vi "CastByteArrayAndDispatchMsg.vi"(8 "error in (no error)":errorcluster, 10 "Raw Data":i8[](array[numeric]), 11 "DIMDemoClient in":refnum<class "DIMDemoClient.lvclass">) -> (0 "error out":errorcluster, 3 "DIMDemoClient out":refnum<class "DIMDemoClient.lvclass">)   [LabVIEW 2012, in "DimActorDemo.lvlib" / "DIMDemoClient.lvclass"]
doc: "Type cast byte array to G data with respect to type descriptor and dispatch message to self.\n\n<b>Needs to be overwitten by derived class.</b>"
uses:
  DIMDemoClient.lvclass
  <vilib>/ActorFramework/Actor/Actor.lvclass/Actor.ctl
  <vilib>/ActorFramework/Message Enqueuer/Message Enqueuer.lvclass/Message Enqueuer.ctl
  DIMDemoClient Messages/Update DemoService Msg/UpdateGUI DemoService Msg.lvclass/UpdateGUI DemoService Msg.ctl
  <vilib>/ActorFramework/Message Enqueuer/Init from Existing Queue.vi
  <vilib>/ActorFramework/Message Enqueuer/Enqueue.vi
  <vilib>/ActorFramework/Message Priority Queue/Priority Enqueue.vi
  <vilib>/ActorFramework/Message Enqueuer/Message Enqueuer.lvclass
  DIMDemoClient Messages/Update DemoService Msg/UpdateGUI DemoService Msg.lvclass
  <vilib>/ActorFramework/Actor/Actor.lvclass
  SVN/LV2009/GPL/lib.lib/DimLVEvent/LVDimInterface/LVDimInterface.lvlib
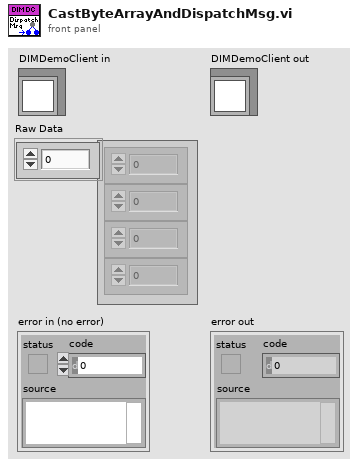
[diagram p1: front panel]
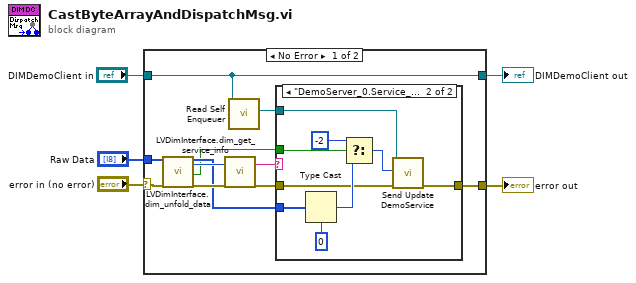
[diagram p0: block diagram]
diagram:
  n1 = case shown="No Error" "error in (no error)" {
    selector: "error in (no error)" -> [w7 w28]
    tunnel: "Raw Data" -> [w9 _]
    tunnel: [w8 w28] -> w4
    tunnel: "DIMDemoClient in" -> [w6 w27]
    tunnel: [w6 w27] -> w1
    frame No Error {
      n2 = call "LVDimInterface.dim_unfold_data.vi"("rawData"=w9, "error in (no error)"=w7) -> ("data"=w13:i8[], "callBackID"=w16:i32, "no link"=w10:bool, "error out"=w15:errorcluster)  [unwired: 14 in]
      n3 = call "LVDimInterface.dim_get_service_info.vi"("callBackID"=w16, "error in (no error)"=w15) -> ("serviceName"=w14:string, "error out"=w11:errorcluster)  [unwired: 8 in, 8 out]
      n4 = call <vilib>:"Read Self Enqueuer.vi"("Actor"=w6) -> ("Self Enqueuer"=w12:refnum<class "Message Enqueuer.lvclass">)  [unwired: 10 in]
      n5 = case shown="\"DemoServer_0.Service_0\"" w14 {
        tunnel: w13 -> [_ w25]
        tunnel: w12 -> [_ w19]
        tunnel: w11 -> [w17 w20]
        tunnel: w10 -> [_ w24]
        tunnel: [w17 w21] -> w8
        frame Default {
        }
        frame "DemoServer_0.Service_0" {
          n6 = Type Cast(type=0, x=w25) -> (*(type *) &x=w22:i32)
          n7 = Select(t=-2, s=w24, f=w22) -> (s? t:f=w18:i32)
          n8 = call "Send Update DemoService.vi"("error in (no error)"=w20, "DemoService"=w18, "Message Enqueuer"=w19) -> ("error out"=w21:errorcluster)  [unwired: 7 in, 1 out]
        }
      }
    }
    frame Error {
    }
  }
  "error out" <- w4
  "DIMDemoClient out" <- w1
